vi "Agilent 87XX Series Read and Graph Data.vi"() -> ()   [LabVIEW 2018]
doc: "This is a simple example VI for the HP8753B Network Analyzer. The VI first recalls a saved state and a saved calibration. It then sets the format to the format shown in \"display 1\" and reads and graphs and the data. It then sets the format the the format shown in \"display 2\" and reads and graphs the data. The data from each display is written to a data file specified in \"output file 1 name\" and \"output file 2 name\".\n\n Some sample files should have been included with this library. These are s{cal,sta,dt1,dt2). All of these were generated with B models. If you are not using a B model, these will probably not work. You can however make your own very easily with \"save/recall state\" and \"save/recall calibration\".\n \n This VI will not work without a saved state and calibration!!!"
uses:
  Agilent 87XX Series.lvlib
panel:
  in  "instrument descriptor (GPIB::16)":string="GPIB::16"
  in  "saved data comments":string="This is a sample output file."
  in  "saver's name":string="Nick Adams"
  out "error out":errorcluster
  in  "display 2":u16(ring)=1 items=["log magnitude", "phase", "delay", "Smith chart", "polar", "linear magnitude", "standing wave ratio", "real", "imaginary"]
  out "graphical display 2":cluster{dbl, dbl}[](graph)
  in  "output file 2 name (read description)":path
  in  "output file 1 name (read description)":path
  in  "calibration file name (read description)":path
  in  "display 1":u16(ring) items=["log magnitude", "phase", "delay", "Smith chart", "polar", "linear magnitude", "standing wave ratio", "real", "imaginary"]
  out "graphical display 1":cluster{dbl, dbl}[](graph)
  in  "state file name (read description)":path
  # "© 2005 National Instruments.  ALL RIGHTS RESERVED."
  # "This VI will not work \nwithout a saved state \nand a saved calibration!!!"
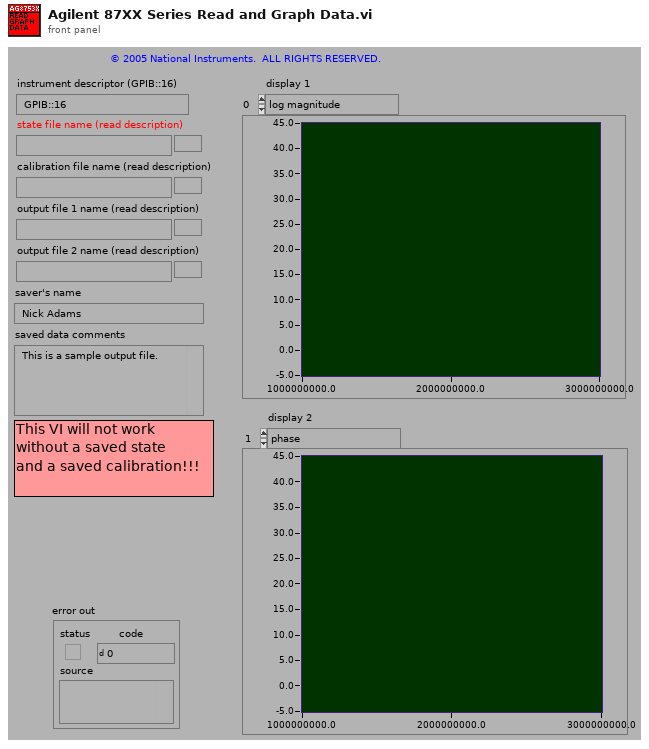
[diagram p1: front panel]
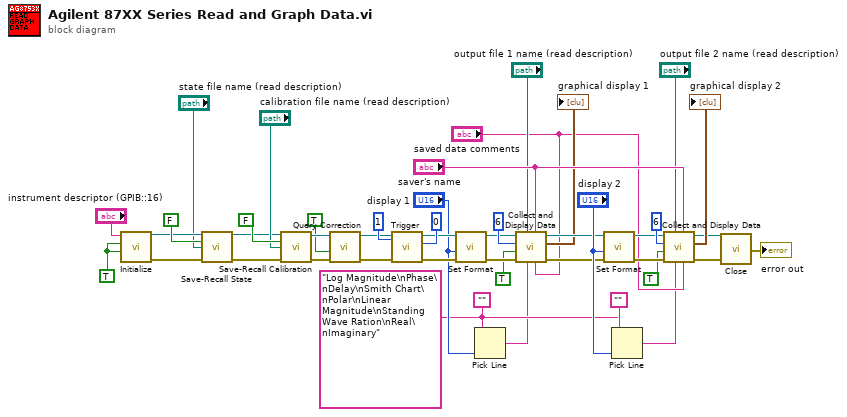
[diagram p0: block diagram]
diagram:
  w27 = TRUE
  w6 = "Log Magnitude\nPhase\nDelay\nSmith Chart\nPolar\nLinear Magnitude\nStanding Wave Ration\nReal\nImaginary"
  n1 = call "Initialize.vi"("reset"=w27, "ID query"=w27, "VISA resource name"="instrument descriptor (GPIB::16)") -> ("error out"=w45:errorcluster, "VISA resource name out"=w35:refnum<visa-resource-name>)  [unwired: 7 in]
  n2 = call "Save-Recall State.vi"("VISA resource name"=w35, "save/recall (f : recall)"=FALSE, "file name (read description)"="state file name (read description)", "error in (no error)"=w45) -> ("VISA resource name out"=w26:refnum<visa-resource-name>, "error out"=w43:errorcluster)  [unwired: 5 in, 5 out]
  n3 = call "Save-Recall Calibration.vi"("VISA resource name"=w26, "save/recall (f : recall)"=FALSE, "file name (read description)"="calibration file name (read description)", "error in (no error)"=w43) -> ("VISA resource name out"=w12:refnum<visa-resource-name>, "error out"=w11:errorcluster)  [unwired: 5 in, 5 out]
  n4 = call "Query Correction.vi"("error in (no error)"=w11, "error message (f : no error)"=TRUE, "VISA resource name"=w12) -> ("error out"=w10:errorcluster, "VISA resource name out"=w13:refnum<visa-resource-name>)  [unwired: 6 in, 1 out]
  n5 = call "Trigger.vi"("trigger (1 : single)"=u16 1, "error in (no error)"=w10, "trigger source (0 : ext trig off)"=u16 0, "VISA resource name"=w13) -> ("error out"=w41:errorcluster, "VISA resource name out"=w25:refnum<visa-resource-name>)  [unwired: 6 in]
  n6 = call "Set Format.vi"("error in (no error)"=w41, "format (0 : log mag)"="display 1", "VISA resource name"=w25) -> ("error out"=w39:errorcluster, "VISA resource name out"=w18:refnum<visa-resource-name>)  [unwired: 7 in]
  n7 = Pick Line(string ("")="", multi-line string=w6, line index="display 1") -> (output string=w5:string)
  n8 = call "Collect and Display Data.vi"("saved data comments"="saved data comments", "saver's name"="saver's name", "saved data title"=w5, "file name (read description)"="output file 1 name (read description)", "error in (no error)"=w39, "save to file"=TRUE, "data type (6 : formatted data)"=u16 6, "VISA resource name"=w18) -> ("error out"=w21:errorcluster, "graphical display"=→"graphical display 1":cluster{dbl, dbl}[], "VISA resource name out"=w22:refnum<visa-resource-name>)  [unwired: 1 out]
  n9 = call "Set Format.vi"("error in (no error)"=w21, "format (0 : log mag)"="display 2", "VISA resource name"=w22) -> ("error out"=w34:errorcluster, "VISA resource name out"=w20:refnum<visa-resource-name>)  [unwired: 7 in]
  n10 = Pick Line(string ("")="", multi-line string=w6, line index="display 2") -> (output string=w3:string)
  n11 = call "Collect and Display Data.vi"("saved data comments"="saved data comments", "saver's name"="saver's name", "saved data title"=w3, "file name (read description)"="output file 2 name (read description)", "error in (no error)"=w34, "save to file"=TRUE, "data type (6 : formatted data)"=u16 6, "VISA resource name"=w20) -> ("error out"=w8:errorcluster, "graphical display"=→"graphical display 2":cluster{dbl, dbl}[], "VISA resource name out"=w2:refnum<visa-resource-name>)  [unwired: 1 out]
  n12 = call "Close.vi"("error in (no error)"=w8, "VISA resource name"=w2) -> ("error out"=→"error out":errorcluster)  [unwired: 9 in]
